vi "ma_Export Signal (CDB).vi"(6 "complex Hann spectrum":cdb[](array[numeric]), 8 "f0":dbl, 9 "export signals":T2(ring), 10 "multiple tone information":T3(array[cluster]) {"detected phase (deg)" format="%_6g"; "detected amplitude" format="%_6p"; "detected frequency" format="%_6p"}, 11 "time signal in":waveform(cdb)) -> (3 "exported signals":T1 {"exported spectrum (dB)"."dB Spectrum (Hann)" format="%.2p"; "exported spectrum (dB)"."df" format="%.2p"; "exported spectrum (dB)"."f0" format="%.2p"})   [LabVIEW 2020, in "NI_MAPro.lvlib"]
uses:
  NI_MAPro.lvlib
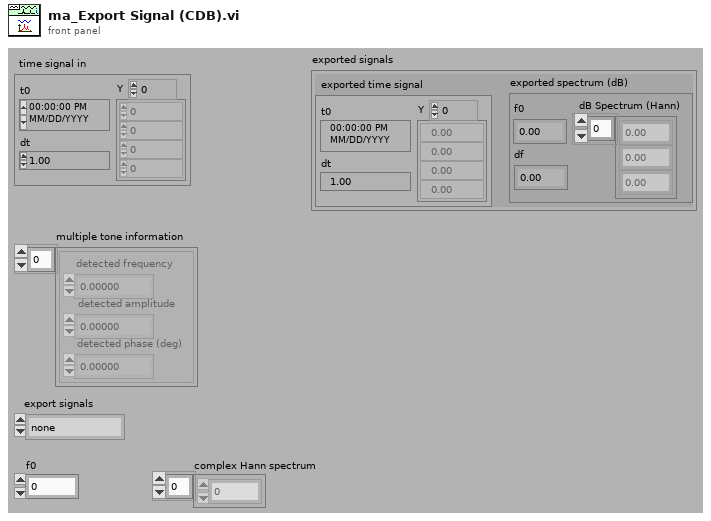
[diagram p1: front panel]
types:
  T1 = cluster{"exported time signal":waveform(cdb), "exported spectrum (dB)":cluster{"f0":dbl, "df":dbl, "dB Spectrum (Hann)":dbl[]}}
  T2 = enum32{"none", "input signal", "detected signal", "residual signal"}
  T3 = cluster{"detected frequency":dbl, "detected amplitude":dbl, "detected phase (deg)":dbl}[]
  T4 = cluster{"f0":dbl, "df":dbl, "dB Spectrum (Hann)":dbl[]}
  T5 = cluster{waveform(dbl), "exported spectrum (dB)":cluster{"f0":dbl, "df":dbl, "dB Spectrum (Hann)":dbl[]}}
  T6 = cluster{"time signal in":waveform(cdb), cluster{"f0":dbl, dbl, dbl[]}}
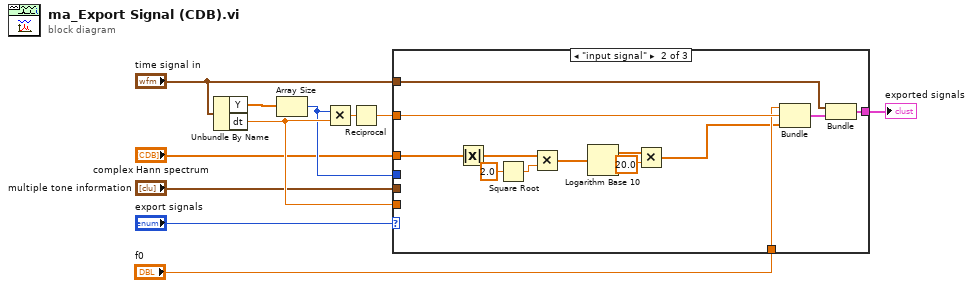
[diagram p0: block diagram]
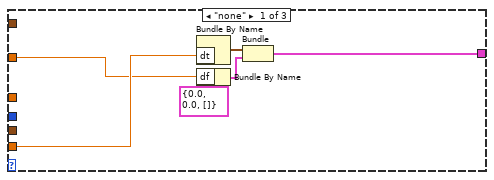
[diagram p2: hidden frame]
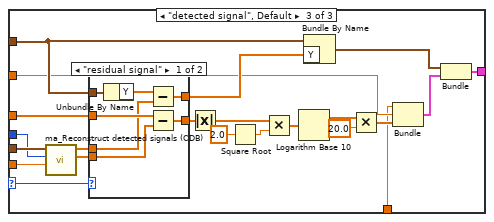
[diagram p3: hidden frame]
diagram:
  n1 = Unbundle By Name("time signal in") -> ("Y"=w6:cdb[], "dt"=w10:dbl)
  n2 = Array Size(array=w6) -> (size(s)=w2:i32)
  n3 = Multiply(x=w2, y=w10) -> (x*y=w9:dbl)
  n4 = Reciprocal(x=w9) -> (1/x=w8:dbl)
  n5 = case shown="\"input signal\"" "export signals" {
    selector: "export signals" -> [_ _ w52]
    tunnel: [w14 w30 w42] -> w7
    tunnel: w10 -> [w13 _ w39]
    tunnel: w8 -> [w12 w25 w43]
    tunnel: "time signal in" -> [_ w29 w45]
    tunnel: "complex Hann spectrum" -> [_ w23 w51]
    tunnel: "f0" -> [_ w24 w36]
    tunnel: "multiple tone information" -> [_ _ w41]
    tunnel: w2 -> [_ _ w40]
    frame "none" {
      n6 = Bundle By Name("dt"=w13) -> (w17:waveform(dbl))  [unwired: 1 out]
      n7 = Bundle By Name(cluster=T4 {"f0"=0.0, "df"=0.0, "dB Spectrum (Hann)"=[]} ("exported spectrum (dB)"), "df"=w12) -> (w15:T4)
      n8 = Bundle(w17, "exported spectrum (dB)"=w15) -> (w14:T5)  [unwired: 1 out]
    }
    frame "input signal" {
      n9 = Absolute Value(x=w23) -> (abs(x)=w20:dbl[])
      n10 = Square Root(x=2.0) -> (sqrt(x)=w21:dbl)
      n11 = Multiply(x=w20, y=w21) -> (x*y=w19:dbl[])
      n12 = Logarithm Base 10(1:w19) -> (0:w28:dbl[])
      n13 = Multiply(x=w28, y=20.0) -> (x*y=w18:dbl[])
      n14 = Bundle("f0"=w24, w25, w18) -> (w26:cluster{"f0":dbl, dbl, dbl[]})  [unwired: 1 out]
      n15 = Bundle("time signal in"=w29, w26) -> (w30:T6)  [unwired: 1 out]
    }
    frame "detected signal", Default {
      n16 = call "ma_Reconstruct detected signals (CDB).vi"("dt"=w39, "# samples"=w40, "multiple tone information"=w41) -> ("complex Hann spectrum"=w38:cdb[], "detected time array"=w37:cdb[])  [unwired: 7 out]
      n17 = case shown="\"residual signal\"" w52 {
        tunnel: [w56 w61] -> w35
        tunnel: w45 -> [w59 _]
        tunnel: [w57 w60] -> w46
        tunnel: w51 -> [w55 _]
        tunnel: w38 -> [w54 w61]
        tunnel: w37 -> [w53 w60]
        frame "residual signal" {
          n18 = Unbundle By Name(w59) -> ("Y"=w58:cdb[])
          n19 = Subtract(x=w58, y=w53) -> (x-y=w57:cdb[])
          n20 = Subtract(x=w55, y=w54) -> (x-y=w56:cdb[])
        }
        frame "detected signal", Default {
        }
      }
      n21 = Absolute Value(x=w35) -> (abs(x)=w32:dbl[])
      n22 = Square Root(x=2.0) -> (sqrt(x)=w34:dbl)
      n23 = Multiply(x=w32, y=w34) -> (x*y=w31:dbl[])
      n24 = Logarithm Base 10(1:w31) -> (0:w50:dbl[])
      n25 = Bundle By Name(cluster=w45, "Y"=w46) -> (w44:waveform(cdb))
      n26 = Multiply(x=w50, y=20.0) -> (x*y=w47:dbl[])
      n27 = Bundle("f0"=w36, w43, w47) -> (w48:cluster{"f0":dbl, dbl, dbl[]})  [unwired: 1 out]
      n28 = Bundle("time signal in"=w44, w48) -> (w42:T6)  [unwired: 1 out]
    }
  }
  "exported signals" <- w7
